vi "getRecordedImageCount.vi"(0 "Camera in":refnum<class "Camera.lvclass">, 11 "error in (no error)":errorcluster) -> (4 "Camera out":refnum<class "Camera.lvclass">, 6 "recorded_image_count":u32, 15 "error out":errorcluster)   [LabVIEW 2019, in "Camera.lvclass"]
doc: "Retreive the rec handle.\nThis handle allows direct access to all underlying functions of the pco.recorder."
uses:
  Camera.lvclass
  pco.recorder/Recorder.lvlib
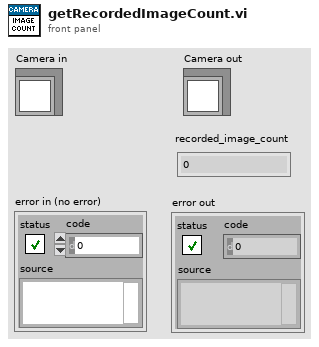
[diagram p1: front panel]
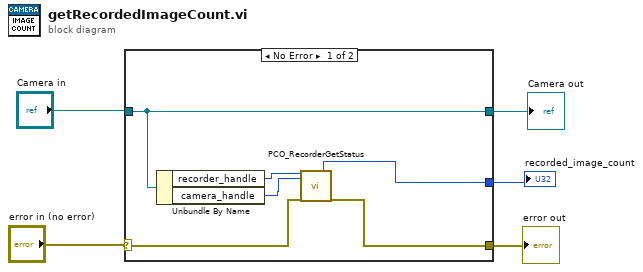
[diagram p0: block diagram]
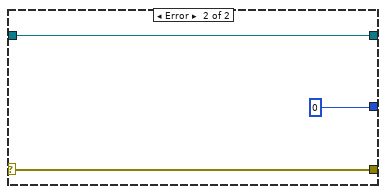
[diagram p2: hidden frame]
diagram:
  n1 = case shown="No Error" "error in (no error)" {
    selector: "error in (no error)" -> [w8 w14]
    tunnel: [w7 w14] -> w3
    tunnel: [w11 w13] -> w4
    tunnel: "Camera in" -> [w11 w13]
    tunnel: [w6 u32 0 ("dwProcImgCount")] -> w1
    frame No Error {
      n2 = Unbundle By Name(w11) -> ("recorder_handle"=w10:u64, "camera_handle"=w9:u64)
      n3 = call "PCO_RecorderGetStatus.vi"("phRec"=w10, "phCam"=w9, "error in (no error)"=w8) -> ("dwProcImgCount"=w6:u32, "error out"=w7:errorcluster)  [unwired: 5 in, 10 out]
    }
    frame Error {
    }
  }
  "error out" <- w3
  "Camera out" <- w4
  "recorded_image_count" <- w1
